vi "assemble images.vi"(6 "bidi_y":bool, 7 "bidi_x":bool, 8 "y pixels":i32=200 min=2 max=1024 step=1, 9 "bin factor":dbl, 10 "x pixels":i32=200 min=2 max=1024 step=1, 11 "raw data in (negative 11 bit data)":i16[](array[numeric])) -> (2 "second image":dbl[][](array[numeric]), 3 "first image":dbl[][](array[numeric]))   [LabVIEW 2012]
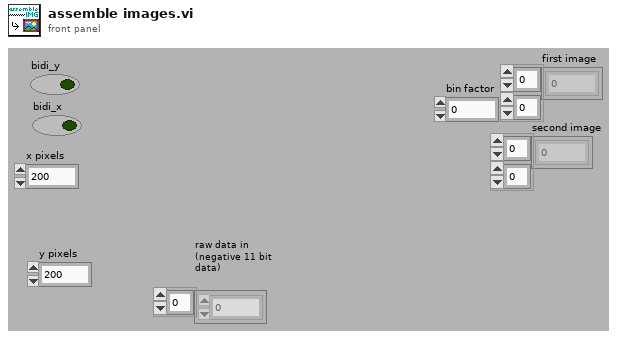
[diagram p1: front panel]
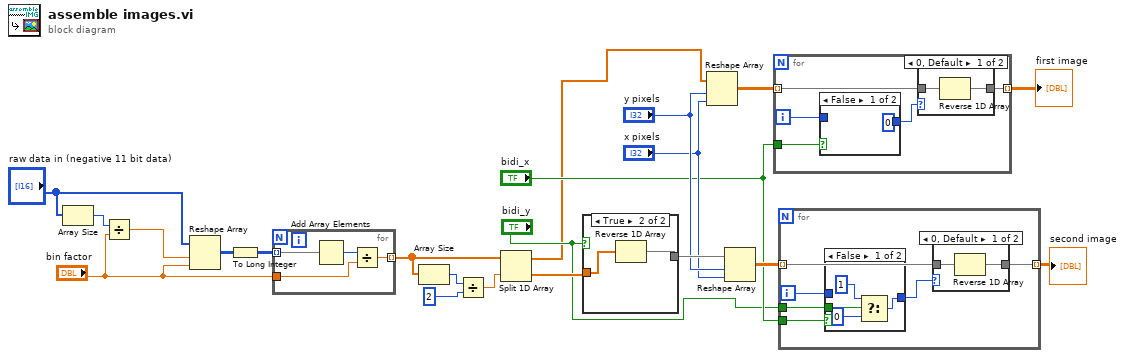
[diagram p0: block diagram]
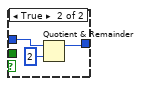
[diagram p3: hidden frame]
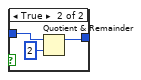
[diagram p5: hidden frame]
diagram:
  n1 = Array Size(array="raw data in (negative 11 bit data)") -> (size(s)=w7:i32)
  n2 = Divide(x=w7, y="bin factor") -> (x/y=w21:dbl)
  n3 = Reshape Array("raw data in (negative 11 bit data)", w21, "bin factor") -> (w20:i16[][])
  n4 = To Long Integer(number=w20) -> (32bit integer=w19:i32[][])
  n5 = for {
    tunnel: w19 -> [w24] mode=indexing
    tunnel: [w23] -> w14 mode=indexing
    tunnel: "bin factor" -> [w22]
    n6 = Add Array Elements(numeric array=w24) -> (sum=w25:i32)
    n7 = Divide(x=w25, y=w22) -> (x/y=w23:dbl)
  }
  n8 = Array Size(array=w14) -> (size(s)=w18:i32)
  n9 = Divide(x=w18, y=2) -> (x/y=w11:dbl)
  n10 = Split 1D Array(array=w14, index=w11) -> (first subarray=w1:dbl[], second subarray=w16:dbl[])
  n11 = case shown="True" "bidi_y" {
    tunnel: w16 -> [w26 w28]
    tunnel: [w26 w27] -> w15
    frame False {
    }
    frame True {
      n12 = Reverse 1D Array(array=w28) -> (reversed array=w27:dbl[])
    }
  }
  n13 = Reshape Array(w1, "y pixels", "x pixels") -> (w13:dbl[][])
  n14 = Reshape Array(w15, "y pixels", "x pixels") -> (w4:dbl[][])
  n15 = for {
    tunnel: w13 -> [w31] mode=indexing
    tunnel: [w30] -> w12 mode=indexing
    tunnel: "bidi_x" -> [w29]
    i -> [w33]
    n16 = case shown="False" w29 {
      tunnel: w33 -> [_ w37]
      tunnel: [0 w35] -> w32
      frame False {
      }
      frame True {
        n17 = Quotient & Remainder(x=w37, y=2) -> (x-y*floor(x/y)=w35:i32)  [unwired: 1 out]
      }
    }
    n18 = case shown="0, Default" w32 {
      tunnel: w31 -> [w39 w40]
      tunnel: [w38 w40] -> w30
      frame 0, Default {
        n19 = Reverse 1D Array(array=w39) -> (reversed array=w38:dbl[])
      }
      frame 1 {
      }
    }
  }
  "first image" <- w12
  n20 = for {
    tunnel: w4 -> [w44] mode=indexing
    tunnel: [w43] -> w5 mode=indexing
    tunnel: "bidi_x" -> [w42]
    tunnel: "bidi_y" -> [w41]
    i -> [w46]
    n21 = case shown="False" w42 {
      tunnel: w46 -> [_ w56]
      tunnel: [w51 w54] -> w45
      tunnel: w41 -> [w52 _]
      frame False {
        n22 = Select(t=1, s=w52, f=0) -> (s? t:f=w51:i32)
      }
      frame True {
        n23 = Quotient & Remainder(x=w56, y=2) -> (x-y*floor(x/y)=w54:i32)  [unwired: 1 out]
      }
    }
    n24 = case shown="0, Default" w45 {
      tunnel: w44 -> [w48 w49]
      tunnel: [w47 w49] -> w43
      frame 0, Default {
        n25 = Reverse 1D Array(array=w48) -> (reversed array=w47:dbl[])
      }
      frame 1 {
      }
    }
  }
  "second image" <- w5
